vi "SENS_CORR_EXT_PORT_INCL_STAT.vi"(0 "VISA IN":refnum<visa-resource-name>, 1 "Port":i32, 2 "Frq. and Loss Pair":i32, 3 "Frq. and Loss ON/OFF":bool, 5 "error in":errorcluster, 7 "Channel":i32) -> (14 "VISA Out":refnum<visa-resource-name>, 19 "error out":errorcluster)   [LabVIEW 2018, in "PNA-X.lvlib"]
doc: "SENSe<cnum>:CORRection:EXTension:PORT<pnum>:INCLude<n>:STATe <bool> \n1704\n\n(Read-Write) Sets and returns the ON/OFF state for the use of the Loss and Freq values for the \nspecified port number. \nLearn about Loss Compensation values. \nNote: This command affects ALL measurements on the specified channel. \nParameters \n<cnum> Any existing channel number. If unspecified, value is set to 1 \n<pnum> Port Number that will receive the Freq/Loss settings. If unspecified, value is set to \n1. \n<n> Freq and Loss pair. Choose from 1 or 2. If unspecified, value is set to 1. \n<value> State of Freq and Loss values for port extension. \n0 or OFF Specified Freq and Loss values are OFF \n1 or ON Specified Freq and Loss values are ON \nExamples SENS:CORR:EXT:PORT:INCL 0 \nsense2:correction:extension:port2:include:state on \nQuery Syntax SENSe<cnum>:CORRection:EXTension:PORT<pnum>:INCLude:STATe? \nReturn Type Boolean \nDefault OFF"
uses:
  PNA-X.lvlib
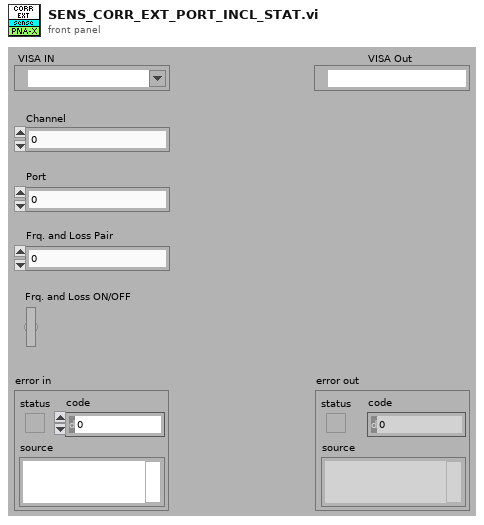
[diagram p1: front panel]
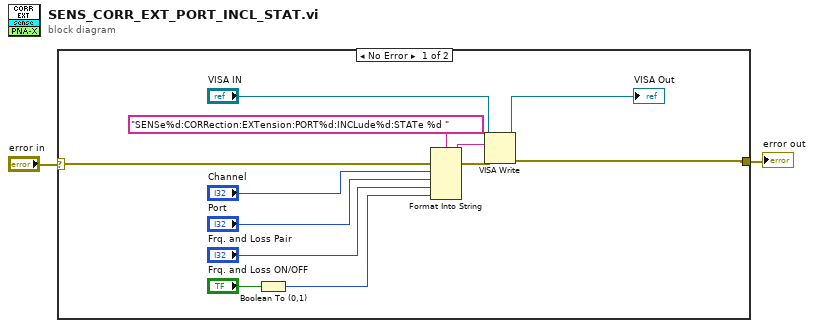
[diagram p0: block diagram]
diagram:
  n1 = case shown="No Error" "error in" {
    selector: "error in" -> [w14 w15]
    tunnel: [w9 w15] -> w1
    frame No Error {
      n2 = Boolean To (0,1)(Boolean="Frq. and Loss ON/OFF") -> (0, 1=w3:i16)
      n3 = Format Into String(format string="SENSe%d:CORRection:EXTension:PORT%d:INCLude%d:STATe %d " ("Cmdline"), error in=w14, "Channel", "Port", "Frq. and Loss Pair", w3) -> (resulting string=w12:string, error out=w13:errorcluster)  [unwired: 1 in]
      n4 = VISA Write(VISA resource name="VISA IN", write buffer=w12, error in (no error)=w13) -> (VISA resource name out=→"VISA Out":refnum<visa-resource-name>, error out=w9:errorcluster)  [unwired: 1 out]
    }
    frame Error {
    }
  }
  "error out" <- w1
